vi "Write Continuous flag.vi"(8 "error in (no error)":errorcluster, 10 "Continuous flag":bool, 11 "Schedule in":refnum<class "Schedule.lvclass">) -> (0 "error out":errorcluster, 3 "Schedule out":refnum<class "Schedule.lvclass">)   [LabVIEW 2020, in "CIRCUS_uServices.lvlib" / "Run Utilities.lvlib" / "Schedule.lvclass"]
uses:
  Schedule.lvclass
  Schedule.lvclass/Schedule.ctl
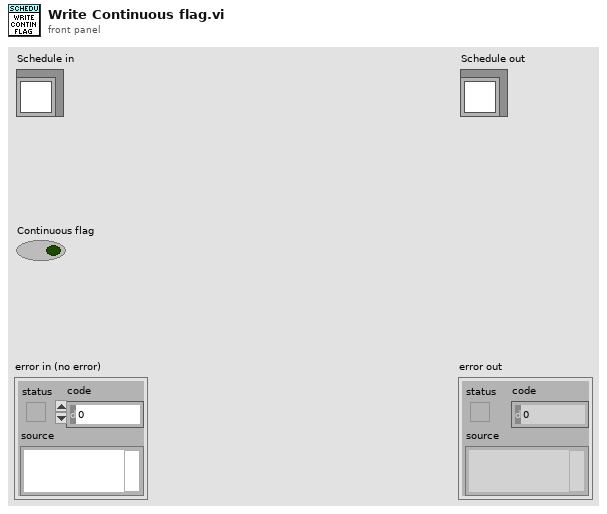
[diagram p1: front panel]
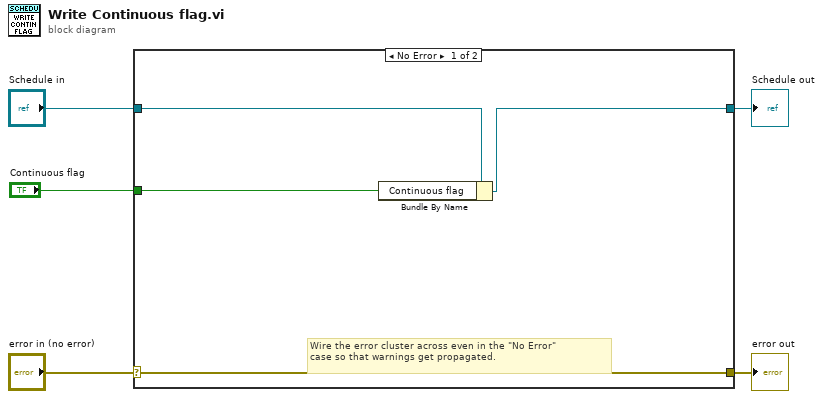
[diagram p0: block diagram]
diagram:
  n1 = case shown="No Error" "error in (no error)" {
    selector: "error in (no error)" -> [w9 w11]
    tunnel: [w9 w11] -> w4
    tunnel: [w7 w10] -> w2
    tunnel: "Schedule in" -> [w8 w10]
    tunnel: "Continuous flag" -> [w6 _]
    frame No Error {
      # "Wire the error cluster across even in the \"No Error\"\ncase so that warnings get propagated."
      n2 = Bundle By Name(cluster=w8, "Continuous flag"=w6) -> (w7:refnum<class "Schedule.lvclass">)
    }
    frame Error {
    }
  }
  "error out" <- w4
  "Schedule out" <- w2
